vi "Temp_EIS.vi"() -> ()   [LabVIEW 2021]
uses:
  <vilib>/Analysis/1siggen.llb/Ramp Pattern by Samples.vi
  c78e2254-4cab-4c10-abc9-ac9a2bb80d81.vi
  c832521a-cced-4df8-9c09-43df9c6be543.vi
  e05b9411-6741-4b16-a09e-be81b5aa145b.vi
  270903f8-5a1e-4e3e-a31f-666567713a2c.vi
  65c142e6-daba-4734-b0d0-1fd8403e1884.vi
  <vilib>/Analysis/baseanly.llb/Mean (DBL).vi
  <vilib>/Utility/file.llb/Write Delimited Spreadsheet (DBL).vi
  C:/Program Files/Metrohm Autolab/Autolab SDK 2.1/EcoChemie.Autolab.Sdk.dll
  EcoChemie.Autolab.Sdk.dll
  <vilib>/Analysis/NI_AALBase.lvlib
panel:
  out "Time (min)":dbl
  out "Bode":cluster{dbl[], dbl[]}[](graph)
  out "Nyquist":cluster{dbl[], dbl[]}(graph)
  out "Data":dbl[][](array[numeric])
  out "Ramp Pattern":dbl[](array[numeric])
  in  "Stop Echem":bool
  out "Heater":bool
  out "Water Temp":dbl
  in  "Sample size":i32=56
  in  "T start":dbl=5.0 format="%0.2f"
  in  "T end":dbl=60.0 format="%0.2f"
  out "Temp LED":bool
  in  "Nox file":path=path "C:/Users/YCL Lab/Documents/NOVA 2.1/Procedures/EIS_FeCN.nox"
  out "Rxn Temp":dbl
  out "Status":string
  out "IsMeasuring":bool
  out "Potentiostat Connected?":bool
  # "Freq, Phase, Z, Z', -Z\""
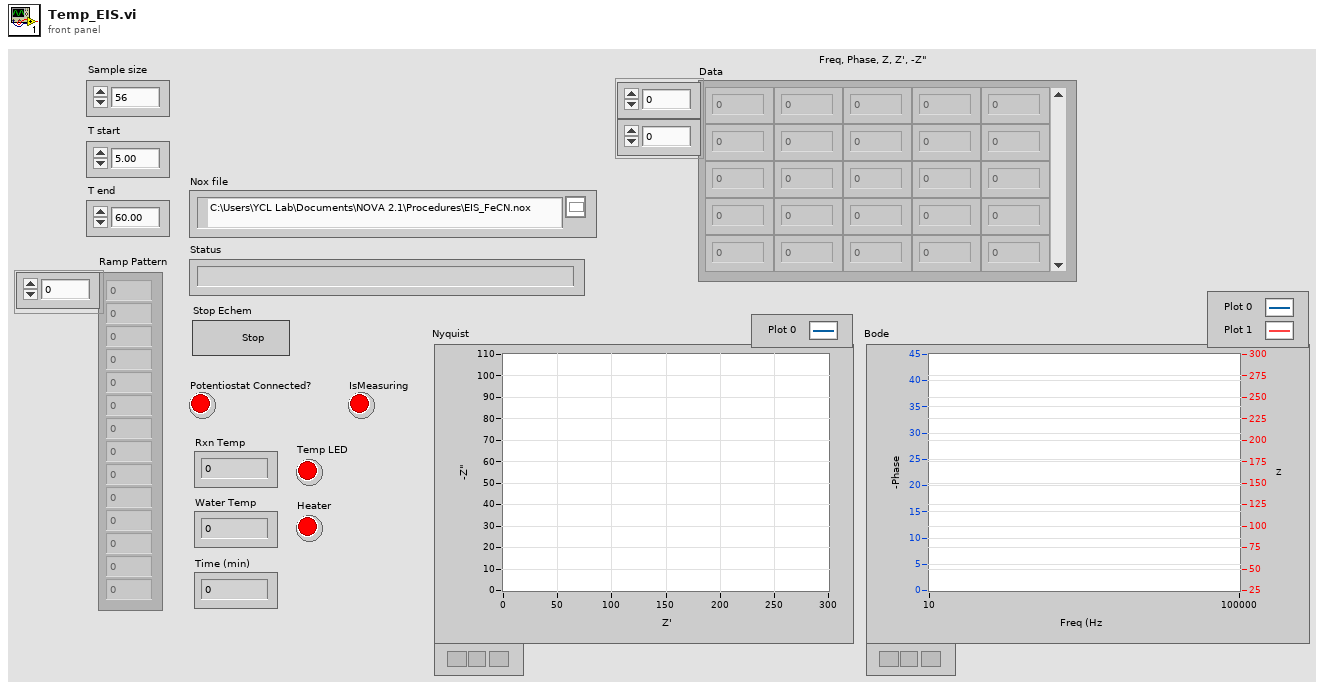
[diagram p1: front panel]
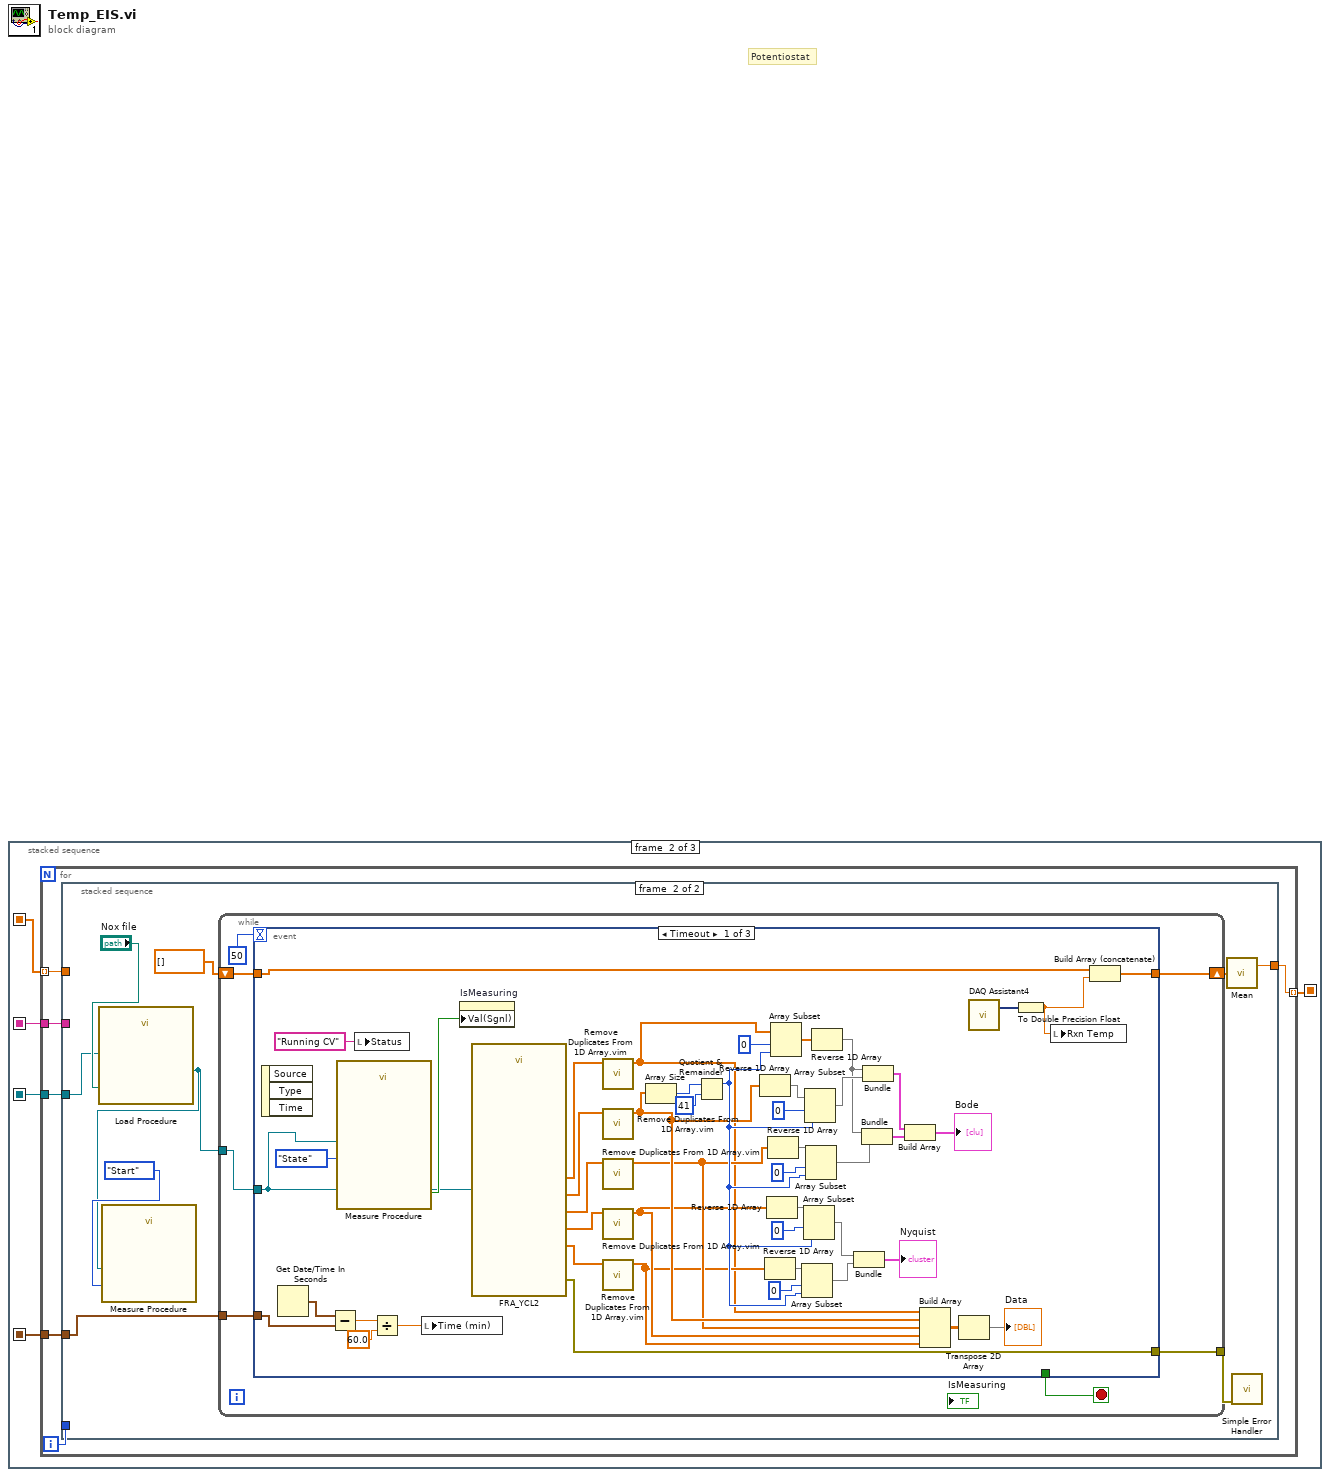
[diagram p0: block diagram]
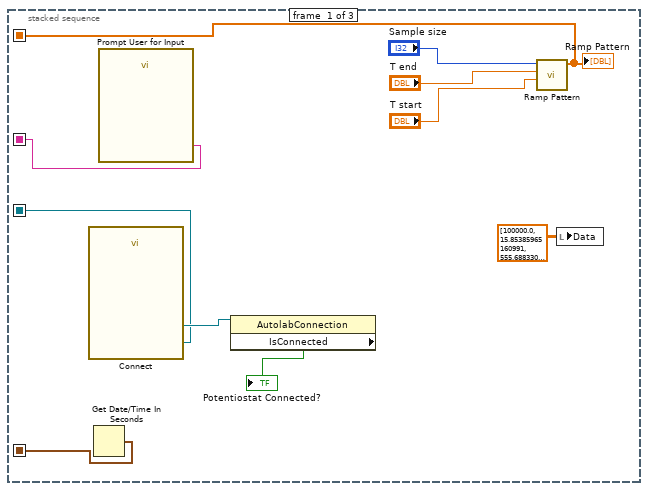
[diagram p2: hidden frame]
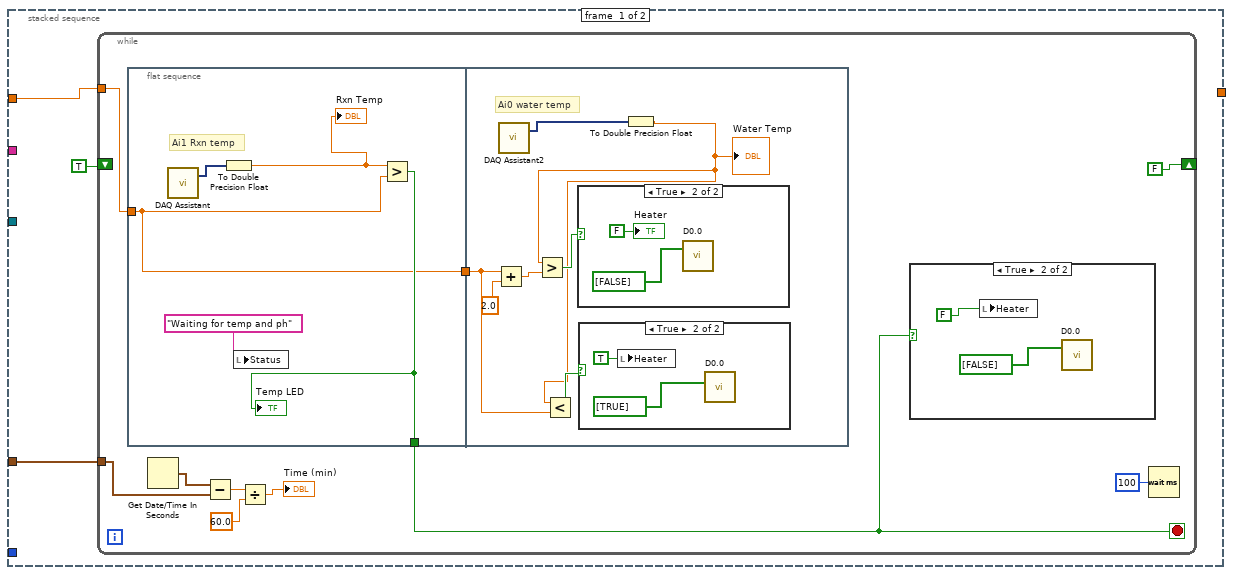
[diagram p3: hidden frame]
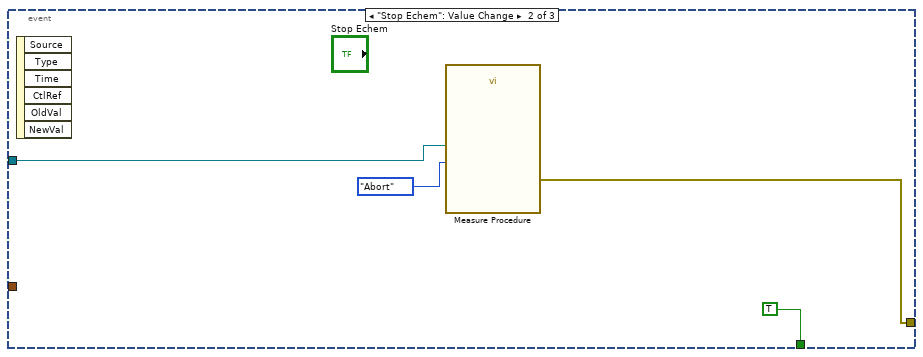
[diagram p7: hidden frame]
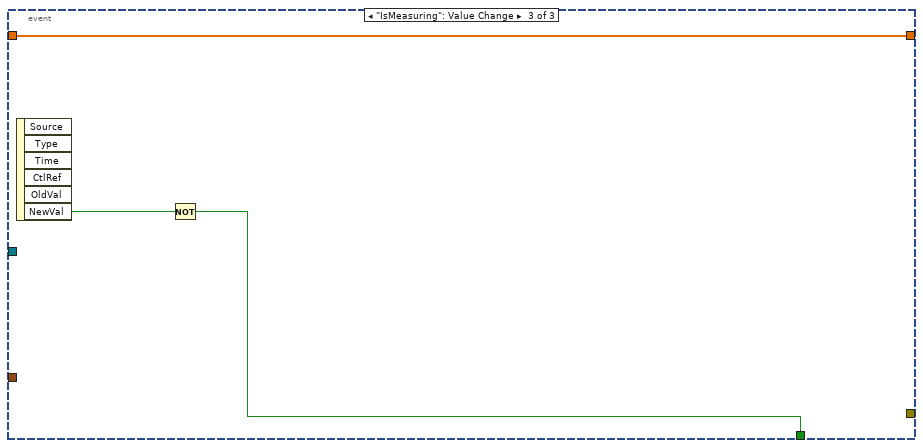
[diagram p8: hidden frame]
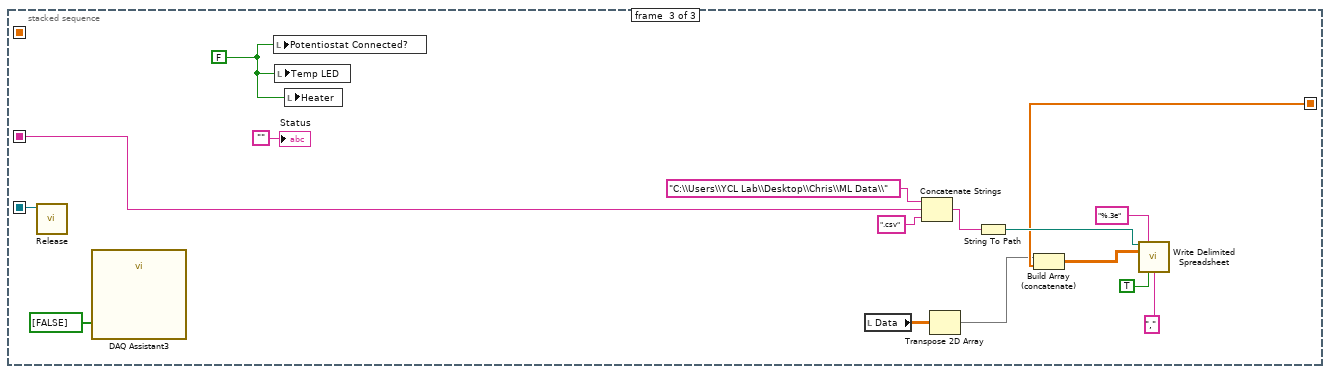
[diagram p9: hidden frame]
diagram:
  # "Potentiostat"
  n1 = stacked-sequence {
    seq-local: [w10 _ _] -> [_ w15 w128]
    seq-local: [w6 _ _] -> [_ w14 _]
    seq-local: [w3 _ _] -> [_ w13 w136]
    seq-local: [_ w12 _] -> [_ _ w126]
    seq-local: [w1 _ _] -> [_ w11 _]
    frame #0 {
      n2 = call "Connect.vi"() -> ("AutolabConnection"=w5:refnum<k24>, "instrument"=w3:refnum<k24>)  [unwired: 8 in, 6 out]
      n3 = Get Date/Time In Seconds() -> (seconds since 1Jan1904=w1:timestamp)
      n4 = call "Prompt User for Input"() -> ("File name"=w10:string)  [unwired: 17 in, 2 out]
      n5 = property class="AutolabConnection"(reference=w5) -> ("IsConnected"=→"Potentiostat Connected?":bool)  [unwired: 1 in, 2 out]
      n6 = call-poly <vilib>:"Ramp Pattern.vi"("start"="T start", "end"="T end", "samples"="Sample size") -> ("Ramp Pattern"=w6:dbl[])  [unwired: 7 in, 1 out]
      "Ramp Pattern" <- w6
      n7 = local write "Data"(dbl[][] [[100000.0, 15.85385965160991, 555.6883303345091, 534.5508449678592, 151.80551575651742], [79433.0, 19.469021219655655, 584.658540027609, 551.2288384718005, 194.86502011455264], [63096.0, 22.96209353248937, 625.4142382360362, 575.8583883232662, 243.98788081806802], [50119.0, 25.995066205695597, 681.9496177212025, 612.9579966261321, 298.89425468244247], [39811.0, 28.198730961734586, 754.665874931708, 665.0975392634323, 356.60320533075327], [31623.0, 29.25412587186114, 843.2342623089148, 735.6888552474203, 412.07515018064373], [25119.0, 29.025838723966856, 944.7603065594516, 826.0993409656669, 458.4014787349619], [19953.0, 27.57635210376669, 1050.1524853017295, 930.8496198545776, 486.147331168225], [15849.0, 25.18035588448757, 1152.9865567614459, 1043.421679741148, 490.5600863490384], [12589.0, 22.22439161591426, 1243.2145247907722, 1150.855681127606, 470.22713221065794], [10000.0, 19.091481603733982, 1317.1609834659387, 1244.7139030262747, 430.81359771722214], [7943.3, 16.083715624999833, 1372.4421340136396, 1318.7219115039459, 380.22352811904193], [6309.6, 13.391647768541667, 1412.1387600946398, 1373.742213916845, 327.05994475703073], [5011.9, 11.094699241350959, 1440.6327591005627, 1413.7080115086153, 277.22266283631456], [3981.1, 9.217452652638087, 1459.565922551298, 1440.7193045326846, 233.79599615878604], [3162.3, 7.7360270457860425, 1471.5961381435407, 1458.2027805082055, 198.0904962816756], [2511.9, 6.6132073206547295, 1480.207626933619, 1470.3586878941983, 170.46978549440092], [1995.3, 5.760509866473373, 1485.7500632435954, 1478.2472094168124, 149.12557889159913], [1584.9, 5.309638262809338, 1489.3323547889702, 1482.9418464560802, 137.81996608144505], [1258.9, 5.085789061300496, 1493.376982137489, 1487.4976809371651, 132.383760275307], [1000.0, 5.119299653867924, 1495.5463123254187, 1489.580676084073, 133.447299512109], [794.33, 5.423011127324958, 1498.4658993234814, 1491.758898629169, 141.6172298698814], [630.96, 6.004624980599655, 1502.0676698109228, 1493.8265071536682, 157.1294091387311], [501.19, 6.889792787894044, 1507.7925348898336, 1496.9043556123158, 180.87475893111085], [398.11, 8.119806266555162, 1516.7165251312065, 1501.511276923403, 214.2262889515029], [316.23, 9.731136069257742, 1530.3916754126863, 1508.372035573884, 258.6744720128875], [251.19, 11.773330882712575, 1550.1768442428438, 1517.5649496641074, 316.29870688587664], [199.53, 14.26805852460944, 1580.9402106907758, 1532.1733887723594, 389.6365697888467], [158.49, 17.214789707553702, 1628.5451660211893, 1555.5895987736312, 481.97547443648637], [125.89, 20.533663559172894, 1700.0125010558118, 1592.0043603148918, 596.2923951254193], [100.0, 24.03485171047112, 1804.831206630288, 1648.3485148936963, 735.0937748847335], [79.433, 27.423046176852548, 1953.1809443000568, 1733.7024047163652, 899.5508729680353], [63.096, 30.296574751463073, 2154.5641776258217, 1860.3061062421884, 1086.9259342689645], [50.119, 32.262034261574144, 2415.7193370143664, 2042.7702561444444, 1289.49199138137], [39.811, 32.98518406283406, 2733.6511800321523, 2293.0177089633717, 1488.2602462175587], [31.623, 32.35291737347772, 3092.045162575883, 2612.060666782277, 1654.654755668941], [25.119, 30.45957996842558, 3471.358507099622, 2992.2658893378166, 1759.7371202308263], [19.953, 27.61364243606853, 3835.9132570481697, 3398.9768094058054, 1777.9727682727391], [15.849, 24.20696262575453, 4159.461751465325, 3793.7215078880067, 1705.5202087606401], [12.589, 20.633074535178665, 4425.418959821312, 4141.556106779647, 1559.4377141592267], [10.0, 17.21155985316881, 4626.182711992143, 4419.016149895113, 1368.8910664114767], [0.0, 15.847523594405613, 555.4922873899128, 534.3790374119611, 151.6928664253641], [0.0, 19.459929692054278, 584.5199976115812, 551.1291240060852, 194.73139520921623], [0.0, 22.95392523152961, 625.5994637656274, 576.063725440787, 243.97801805720565], [0.0, 25.989472456519533, 681.6679073225545, 612.7339522383123, 298.7109633875668], [0.0, 28.19405713534713, 754.4652789962716, 664.9498307573858, 356.4541762788674], [0.0, 29.253694901847897, 843.2763296089014, 735.728657017945, 412.09017377417706], [0.0, 29.026103252852472, 944.3071457690097, 825.7009813374924, 458.18541549106044], [0.0, 27.58042793909113, 1049.9623316919465, 930.6464896664855, 486.12550770705], [0.0, 25.1880377549509, 1152.6970122450905, 1043.0938855988816, 490.57675022873394], [0.0, 22.229680790785427, 1242.7946701030426, 1150.4236190298593, 470.1745301638228], [0.0, 19.09842107672328, 1316.3772735624007, 1243.9211423088539, 430.70792663778], [0.0, 16.09023724317631, 1372.3955533550263, 1318.6338685827918, 380.3607176024219], [0.0, 13.395056159825067, 1412.274342016148, 1373.8546489920777, 327.17307431999814], [0.0, 11.09962626494285, 1440.6093739369128, 1413.6612194141615, 277.33972849083517], [0.0, 9.220767698080829, 1459.5377383790037, 1440.677955061995, 233.8748373615373], [0.0, 7.73820130343692, 1471.7304323039496, 1458.3283335592735, 198.16391424223374], [0.0, 6.616214323022801, 1480.1406496757972, 1470.2832080556532, 170.53923575608042], [0.0, 5.762615493945848, 1486.0520512943133, 1478.5421899681667, 149.2102263257245], [0.0, 5.310337495984809, 1489.4068765020643, 1483.0143662687558, 137.84496077882432], [0.0, 5.08770245988296, 1493.077658360416, 1487.1951146601832, 132.40689115717277], [0.0, 5.121647422412409, 1495.4206033776063, 1489.4499996148068, 133.4971147766728], [0.0, 5.420588605002794, 1498.5367165939697, 1491.8353855941255, 141.56084652707577], [0.0, 6.003824686282847, 1502.5821533643084, 1494.340363323156, 157.16235602758206], [0.0, 6.890837870288462, 1508.2598599360517, 1497.365005526967, 180.95813139382386], [0.0, 8.119912892795302, 1516.4168596398151, 1501.214217016723, 214.18675688927587], [0.0, 9.732392512843017, 1529.8072204810533, 1507.7903192302322, 258.60874902361735], [0.0, 11.77513521356597, 1549.9607147641586, 1517.343406927336, 316.3023913383628], [0.0, 14.268339729034814, 1580.864130321905, 1532.0977429928791, 389.62533856842356], [0.0, 17.21669988690005, 1629.1355859392631, 1556.13749382826, 482.2020921517949], [0.0, 20.530192095504525, 1700.305415314386, 1592.314796383872, 596.2986622192061], [0.0, 24.03519156606299, 1804.7891981222551, 1648.3057884033126, 735.0864422466972], [0.0, 27.426326523651475, 1952.7019090967449, 1733.2257065373346, 899.4294836107105], [0.0, 30.309759700606946, 2155.2016716552366, 1860.6062874639201, 1087.6757276666856], [0.0, 32.260502743205556, 2415.0742856191073, 2042.2592487785082, 1289.0930788105586], [0.0, 32.98595780993021, 2731.988422548931, 2291.602882973172, 1487.3859511540516], [0.0, 32.349211999704934, 3092.3447808416727, 2612.4207877299104, 1654.6461468952705], [0.0, 30.45962644391766, 3471.1443591372254, 2992.0798692548256, 1759.6309891480669], [0.0, 27.62285737733186, 3834.6256306432683, 3397.54995114089, 1777.9223989501963], [0.0, 24.203527180939783, 4158.894524167539, 3793.3063986450643, 1705.0601834390336], [0.0, 20.62275241705541, 4423.766161626665, 4140.290093524926, 1558.1094294729355], [0.0, 17.19984875698757, 4627.116922209654, 4420.188286603359, 1368.2640544768408], [0.0, 15.845401431542403, 555.5166066345568, 534.4080507168308, 151.67971379129816], [0.0, 19.4581148981441, 584.3316335361544, 550.9576859661532, 194.6511911750152], [0.0, 22.95085457889017, 625.5909341541734, 576.0689457225611, 243.94381867550632], [0.0, 25.98552447678983, 681.5704193935925, 612.6669011714542, 298.62602833866487], [0.0, 28.192413989043537, 754.5689609604074, 665.0514347474996, 356.48408938571316], [0.0, 29.253583697024677, 843.0436223283922, 735.5264277777075, 411.97502738532796], [0.0, 29.025401827341174, 944.1853084072064, 825.6000553063419, 458.11619191006196], [0.0, 27.58036273013996, 1050.3049902710263, 930.950762582013, 486.2830968028697], [0.0, 25.188477656537174, 1152.8885404221105, 1043.2634353238361, 490.66627268738597], [0.0, 22.231571860579233, 1242.952808062215, 1150.5544824452606, 470.2723317343509], [0.0, 19.100068404459243, 1316.5202852201314, 1244.0438970395173, 430.79048693631484], [0.0, 16.09056685083661, 1372.2256278009686, 1318.4684117589047, 380.32120738622217], [0.0, 13.395609494426878, 1412.6460158924265, 1374.2130512312897, 327.27244925647904], [0.0, 11.099008605240853, 1440.8842640574976, 1413.9339576829148, 277.37740664957954], [0.0, 9.220703211531193, 1459.282902654721, 1440.4266754413716, 233.83238154136313], [0.0, 7.736081374785574, 1471.9165868204532, 1458.5201248281478, 198.13501464520792], [0.0, 6.615651005725932, 1480.3661849531072, 1470.5089181950889, 170.55076388373791]] ("Data")) -> ()
    }
    frame #1 {
      n8 = for {
        tunnel: w14 -> [w21] mode=indexing
        tunnel: w15 -> [w19]
        tunnel: w13 -> [w18]
        tunnel: [w17] -> w12 mode=indexing
        tunnel: w11 -> [w16]
        i -> [w20]
        n9 = stacked-sequence {
          tunnel: w21 -> [w24 _]
          tunnel: w20 -> [_ _]
          tunnel: w19 -> [_ _]
          tunnel: w18 -> [_ w55]
          tunnel: [_ w54] -> w17
          tunnel: w16 -> [w22 w53]
          frame #0 {
            n10 = while {
              tunnel: w24 -> [w33]
              shift-right: [FALSE] -> _
              shift-left: TRUE -> [_]
              tunnel: w22 -> [w28]
              stop <- w30 stop-if-true
              n11 = flat-sequence {
                tunnel: [w40] -> w30
                tunnel: w33 -> [w38]
                tunnel: [w38] -> w31
                tunnel: w31 -> [w43]
                frame #0 {
                  # "Ai1 Rxn temp"
                  n12 = call "DAQ Assistant"() -> ("data"=w37:dynamicdata)  [unwired: 17 in, 2 out]
                  n13 = To Double Precision Float(number=w37) -> (double precision float=w39:dbl)
                  "Rxn Temp" <- w39
                  n14 = local write "Status"("Waiting for temp and ph" ("Status")) -> ()
                  n15 = Greater?(x=w39, y=w38) -> (0:w40:bool)
                  "Temp LED" <- w40
                }
                frame #1 {
                  # "Ai0 water temp"
                  n16 = Add(x=w43, y=2.0) -> (x+y=w48:dbl)
                  n17 = call "DAQ Assistant2"() -> ("data"=w42:dynamicdata)  [unwired: 17 in, 2 out]
                  n18 = To Double Precision Float(number=w42) -> (double precision float=w44:dbl)
                  "Water Temp" <- w44
                  n19 = Greater?(x=w44, y=w48) -> (0:w46:bool)
                  n20 = Less?(x=w44, y=w43) -> (x < y?=w45:bool)
                  n21 = case shown="True" w46 {
                    frame False {
                    }
                    frame True {
                      n22 = call "D0.0"("data"=bool[] [FALSE]) -> ()  [unwired: 17 in, 2 out]
                      "Heater" <- FALSE ("Heater")
                    }
                  }
                  n23 = case shown="True" w45 {
                    frame False {
                    }
                    frame True {
                      n24 = local write "Heater"(TRUE ("Heater")) -> ()
                      n25 = call "D0.0"("data"=bool[] [TRUE]) -> ()  [unwired: 17 in, 2 out]
                    }
                  }
                }
              }
              n26 = Get Date/Time In Seconds() -> (seconds since 1Jan1904=w29:timestamp)
              n27 = Subtract(x=w29, y=w28) -> (x-y=w27:dbl)
              n28 = Divide(x=w27, y=60.0) -> (x/y=→"Time (min)":dbl)
              n29 = case shown="True" w30 {
                frame False {
                }
                frame True {
                  n30 = local write "Heater"(FALSE ("Heater")) -> ()
                  n31 = call "D0.0"("data"=bool[] [FALSE]) -> ()  [unwired: 17 in, 2 out]
                }
              }
              n32 = Wait (ms)(milliseconds to wait=u32 100) -> ()  [unwired: 1 out]
            }
          }
          frame #1 {
            n33 = call "Load Procedure.vi"("Procedure"="Nox file", "Instrument"=w55) -> ("LoadProcedure"=w56:refnum<k24>)  [unwired: 6 in, 3 out]
            n34 = call "Measure Procedure.vi"("Request for procedure"=enum16{"State", "Save", "Abort", "Start"}."Start", "LoadProcedure"=w56) -> ()  [unwired: 8 in, 2 out]
            n35 = while {
              tunnel: w56 -> [w66]
              tunnel: [w65] -> w59
              shift-right: [w64] -> w58
              shift-left: dbl[] [] -> [w63]
              tunnel: w53 -> [w62]
              stop <- w67 stop-if-true
              n36 = event shown="[0] Timeout" {
                selector: _ -> [_ _ _]
                dyn-events: _ -> [_ _ _]
                timeout: 50 -> [_ _ _]
                tunnel: [_ TRUE w121] -> w67
                tunnel: w66 -> [w109 w120 _]
                tunnel: [w108 w117 _] -> w65
                tunnel: [w113 _ w122] -> w64
                tunnel: w63 -> [w112 _ w122]
                tunnel: w62 -> [w72 _ _]
                event Timeout {
                  n37 = event-data() -> ()  [unwired: 1 in, 3 out]
                  n38 = Get Date/Time In Seconds() -> (seconds since 1Jan1904=w73:timestamp)
                  n39 = Subtract(x=w73, y=w72) -> (x-y=w71:dbl)
                  n40 = call "Measure Procedure.vi"("Request for procedure"=enum16{"State", "Save", "Abort", "Start"}."State", "LoadProcedure"=w109) -> ("IsMeasuring"=w115:bool)  [unwired: 8 in, 1 out]
                  n41 = local write "Status"("Running CV" ("Status")) -> ()
                  n42 = Divide(x=w71, y=60.0) -> (x/y=w70:dbl)
                  n43 = local write "Time (min)"(w70) -> ()
                  n44 = property on="IsMeasuring" class="Bool (strict)"("Val(Sgnl)"=w115) -> ()  [unwired: 2 in, 2 out]
                  n45 = call "FRA_YCL2.vi"("LoadProcedure"=w109) -> ("-Phase"=w107:dbl[], "Frequency"=w103:dbl[], "-Z''"=w106:dbl[], "Z"=w105:dbl[], "Z'"=w104:dbl[], "error out"=w108:errorcluster)  [unwired: 17 in, 4 out]
                  n46 = call "Remove Duplicates From 1D Array.vim"("array"=w103) -> ("array with duplicates removed"=w76:dbl[])  [unwired: 10 in]
                  n47 = call "Remove Duplicates From 1D Array.vim"("array"=w107) -> ("array with duplicates removed"=w84:dbl[])  [unwired: 10 in]
                  n48 = call "Remove Duplicates From 1D Array.vim"("array"=w105) -> ("array with duplicates removed"=w82:dbl[])  [unwired: 10 in]
                  n49 = call "Remove Duplicates From 1D Array.vim"("array"=w104) -> ("array with duplicates removed"=w79:dbl[])  [unwired: 10 in]
                  n50 = call "Remove Duplicates From 1D Array.vim"("array"=w106) -> ("array with duplicates removed"=w77:dbl[])  [unwired: 10 in]
                  n51 = Array Size(array=w84) -> (size(s)=w100:i32)
                  n52 = Quotient & Remainder(x=w100, y=41) -> (x-y*floor(x/y)=w85:i32)  [unwired: 1 out]
                  n53 = Reverse 1D Array(array=w84) -> (reversed array=w83:dbl[])
                  n54 = Reverse 1D Array(array=w77) -> (reversed array=w80:dbl[])
                  n55 = Reverse 1D Array(array=w79) -> (reversed array=w78:dbl[])
                  n56 = Reverse 1D Array(array=w82) -> (reversed array=w81:dbl[])
                  n57 = Array Subset(array=w76, index=0, length=w85) -> (w75:dbl[])
                  n58 = Array Subset(array=w80, index=0, length=w85) -> (w92:dbl[])
                  n59 = Array Subset(array=w78, index=0, length=w85) -> (w93:dbl[])
                  n60 = Array Subset(array=w83, index=0, length=w85) -> (w90:dbl[])
                  n61 = Array Subset(array=w81, index=0, length=w85) -> (w89:dbl[])
                  n62 = Reverse 1D Array(array=w75) -> (reversed array=w74:dbl[])
                  n63 = Bundle(w93, w92) -> (→"Nyquist":cluster{dbl[], dbl[]})  [unwired: 1 in]
                  n64 = Bundle(w74, w89) -> (w88:cluster{dbl[], dbl[]})  [unwired: 1 in]
                  n65 = Bundle(w74, w90) -> (w87:cluster{dbl[], dbl[]})  [unwired: 1 in]
                  n66 = Build Array(w87, w88) -> (→"Bode":cluster{dbl[], dbl[]}[])
                  n67 = Build Array(w76, w84, w82, w79, w77) -> (w102:dbl[][])
                  n68 = Transpose 2D Array(2D array=w102) -> (transposed array=→"Data":dbl[][])
                  n69 = call "DAQ Assistant4"() -> ("data"=w110:dynamicdata)  [unwired: 17 in, 2 out]
                  n70 = To Double Precision Float(number=w110) -> (double precision float=w111:dbl)
                  n71 = local write "Rxn Temp"(w111) -> ()
                  n72 = Build Array (concatenate)(w112, w111) -> (w113:dbl[])
                }
                event "Stop Echem": Value Change {
                  n73 = event-data() -> ()  [unwired: 1 in, 6 out]
                  n74 = call "Measure Procedure.vi"("Request for procedure"=enum16{"State", "Save", "Abort", "Start"}."Abort", "LoadProcedure"=w120) -> ("error out"=w117:errorcluster)  [unwired: 8 in, 1 out]
                }
                event "IsMeasuring": Value Change {
                  n75 = event-data() -> ("NewVal"=w123:bool)  [unwired: 1 in, 5 out]
                  n76 = Not(x=w123) -> (.not. x?=w121:bool)
                }
              }
            }
            n77 = call-poly <vilib>:"Mean.vi"("X"=w58) -> ("mean"=w54:dbl)  [unwired: 1 out]
            n78 = call <vilib>:"Simple Error Handler.vi"("error in (no error)"=w59) -> ()  [unwired: 4 in, 5 out]
          }
        }
      }
    }
    frame #2 {
      w138 = FALSE ("pH LED")
      n79 = call "Release.vi"("Instrument"=w136) -> ()  [unwired: 10 in, 1 out]
      n80 = call "DAQ Assistant3"("data"=bool[] [FALSE]) -> ()  [unwired: 17 in, 2 out]
      n81 = local write "Potentiostat Connected?"(w138) -> ()
      n82 = local write "Temp LED"(w138) -> ()
      n83 = local write "Heater"(w138) -> ()
      n84 = local read "Data"() -> (w125:dbl[][])
      n85 = Concatenate Strings("C:\\Users\\YCL Lab\\Desktop\\Chris\\ML Data\\", w128, ".csv" ("string")) -> (w135:string)
      n86 = Transpose 2D Array(2D array=w125) -> (transposed array=w124:dbl[][])
      n87 = String To Path(string=w135) -> (path=w134:path)
      n88 = Build Array (concatenate)(w124, w126) -> (w127:dbl[][])
      n89 = call-poly <vilib>:"Write Delimited Spreadsheet.vi"("file path (dialog if empty)"=w134, "format (%.3f)"="%.3e", "2D data"=w127, "transpose? (no:F)"=TRUE, "delimiter (\\t)"="," ("delimiter (\\t)")) -> ()  [unwired: 9 in, 2 out]
      "Status" <- ""
    }
  }
